vi "Create.vi"(8 "error in (no error)":errorcluster) -> (0 "error out":errorcluster, 3 "Core Component":refnum<class "Core Component.lvclass">)   [LabVIEW 2017, in "DSF Core.lvlib" / "Core Component.lvclass"]
uses:
  Core Component.lvclass
  C:/Git/DSF/Core/Classes/Component/Component.lvclass
  Component User Interface/Core/Core Component User Interfaces.lvclass
  Component Configuration/Core/Core Component Configurations.lvclass
  Component.lvclass/Component.ctl
  Component Configuration/Find.vi
  Component User Interface/Find.vi
  <vilib>/Utility/error.llb/Clear Errors.vi
  Component Configuration/Component Configurations.lvclass
  Component User Interface/Component User Interfaces.lvclass
  Component.lvclass
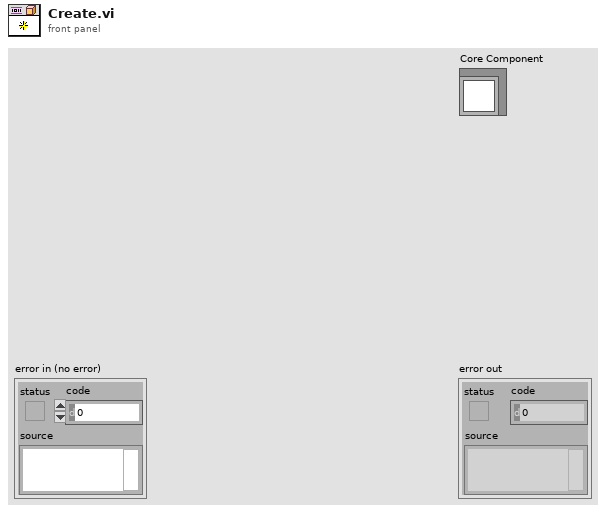
[diagram p1: front panel]
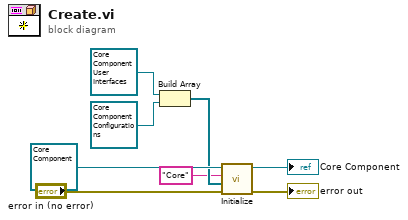
[diagram p0: block diagram]
diagram:
  n1 = Build Array(refnum<class "Core Component User Interfaces.lvclass"> refnum ("DSF Core.lvlib:Core User Interfaces.lvclass"), refnum<class "Core Component Configurations.lvclass"> refnum ("DSF Core.lvlib:Core Configurations.lvclass")) -> (w2:refnum<class>[])
  n2 = call "Initialize.vi"("error in (no error)"="error in (no error)", "objects"=w2, "name"="Core", "Component in"=refnum<class "Core Component.lvclass"> refnum ("Core Component in")) -> ("error out"=→"error out":errorcluster, "Component out"=→"Core Component":refnum<class "Core Component.lvclass">)  [unwired: 6 in]
